vi "programacion 2 tercer parcial.vi"() -> ()   [LabVIEW 2011]
uses:
  Control programacion 2 tercer parcial.ctl
panel:
  out "Array":T1(array[cluster]) {"Velocidad 3" scale=0.0..180.0; "Velocidad 2" scale=0.0..180.0; "Velocidad1" scale=0.0..180.0}
  # "Se tiene que ingresar las tres velocidades de cada elemento del arreglo \nluego se debera de obtener el promedio de cada uno de los elementos del arreglo.\n\nIniciar arreglo, rellenar arreglo, obtener promedio, finalizar."
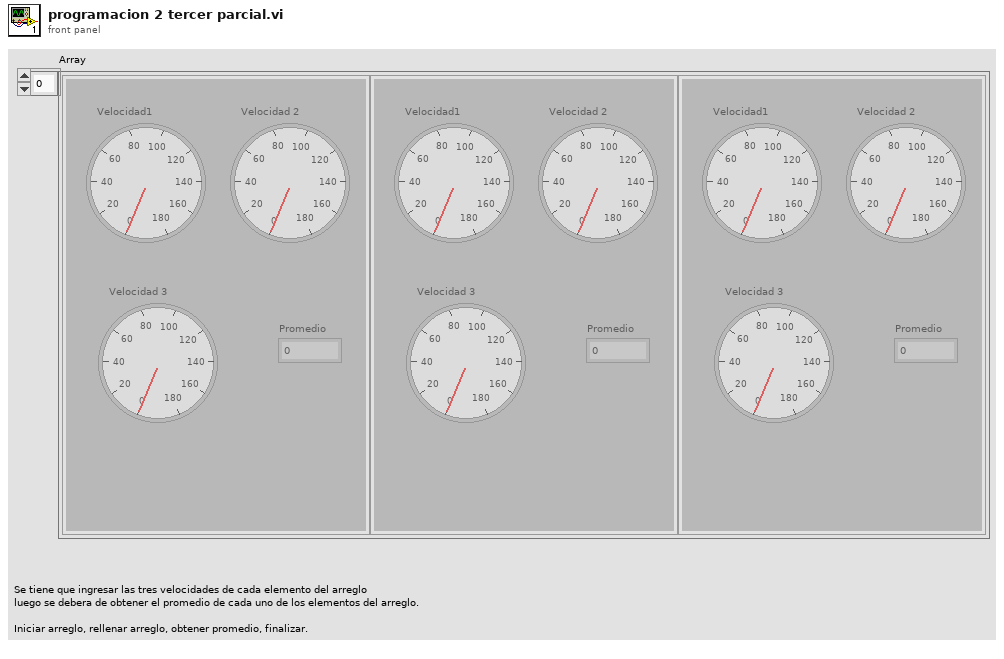
[diagram p1: front panel]
types:
  T1 = cluster{"Velocidad1":i32, "Velocidad 2":i32, "Velocidad 3":i32, "Promedio":dbl}[]
  T2 = typedef "Control programacion 2 tercer parcial.ctl" = enum16{"iniciar arreglo", "rellenar arreglo", "obtener promedio", "finalizar"}
  T3 = cluster{"Velocidad1":i32, "Velocidad 2":i32, "Velocidad 3":i32, "Promedio":dbl}
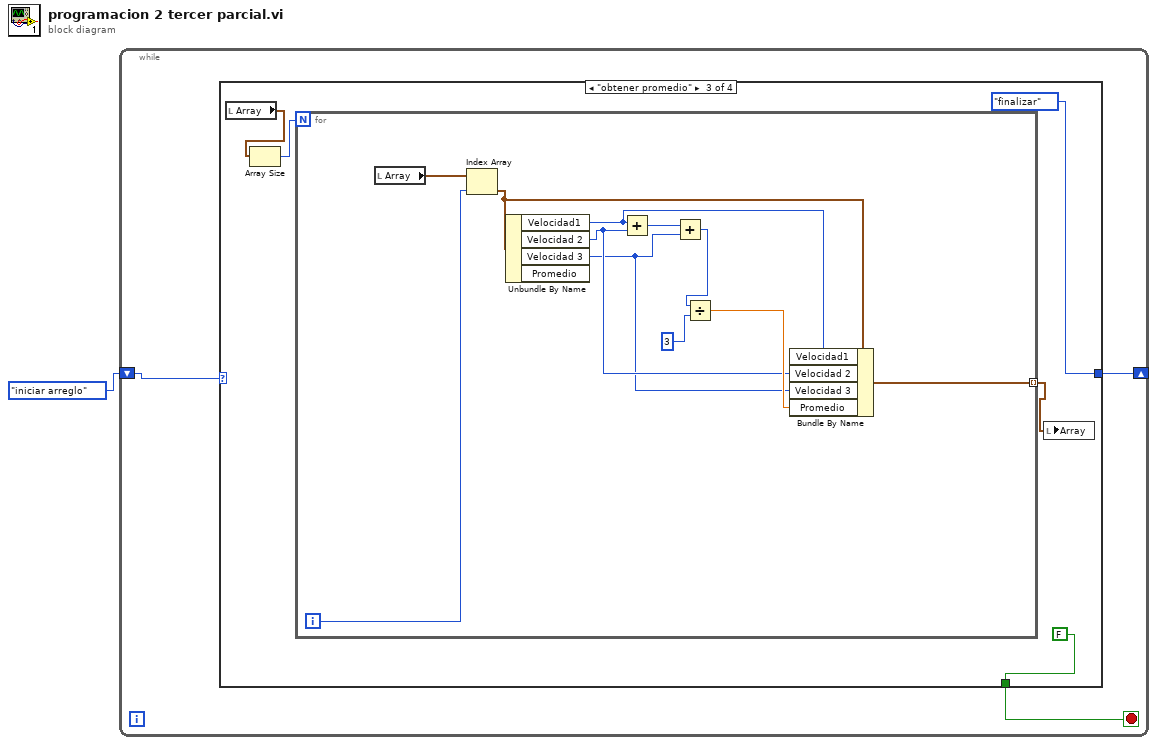
[diagram p0: block diagram]
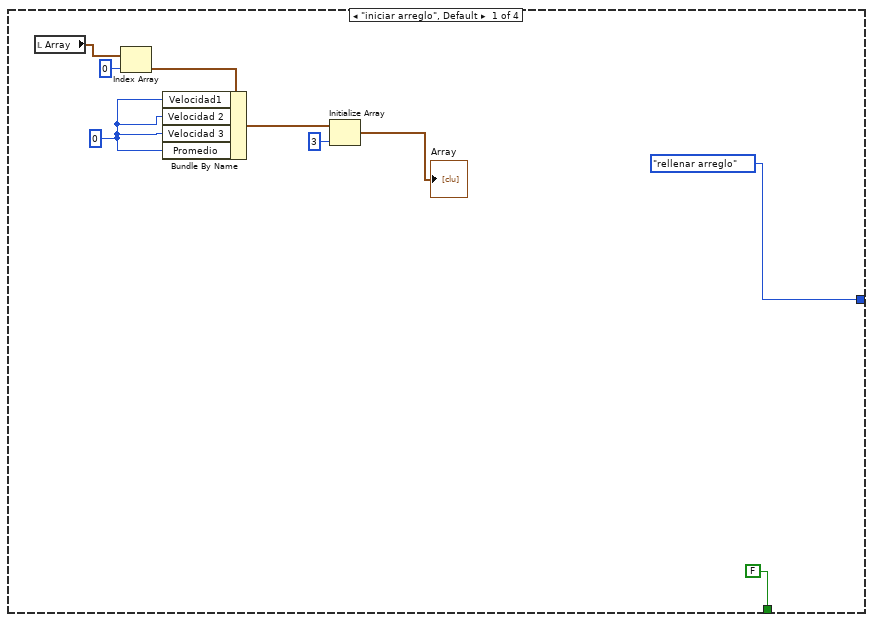
[diagram p2: hidden frame]
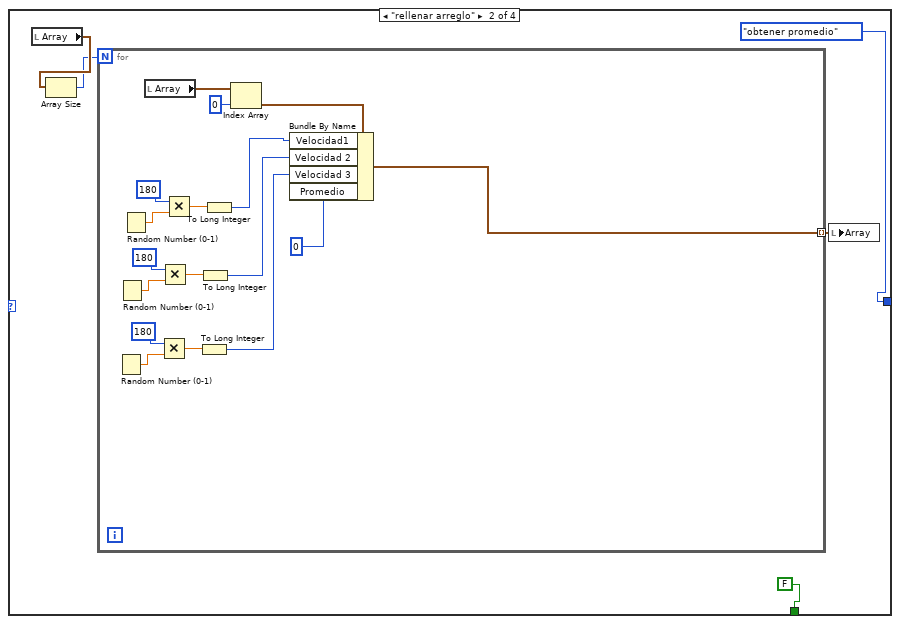
[diagram p3: hidden frame]
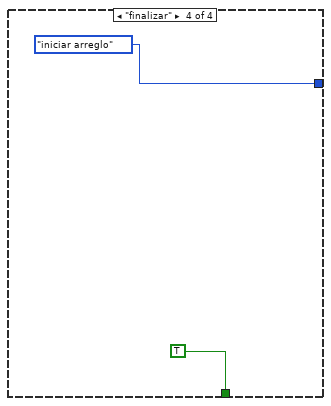
[diagram p4: hidden frame]
diagram:
  n1 = while {
    shift-right: [w3] -> _
    shift-left: Control_programacion_2_tercer_parcial."iniciar arreglo" -> [w4]
    stop <- w2 stop-if-true
    n2 = case shown="\"obtener promedio\"" w4 {
      tunnel: [Control_programacion_2_tercer_parcial."rellenar arreglo" Control_programacion_2_tercer_parcial."obtener promedio" Control_programacion_2_tercer_parcial."finalizar" Control_programacion_2_tercer_parcial."iniciar arreglo"] -> w3
      tunnel: [FALSE FALSE FALSE TRUE] -> w2
      frame "iniciar arreglo", Default {
        w10 = 0
        n3 = local read "Array"() -> (w13:T1)
        n4 = Index Array(array=w13, index=0) -> (element=w11:T3)
        n5 = Bundle By Name(cluster=w11, "Velocidad1"=w10, "Velocidad 2"=w10, "Velocidad 3"=w10, "Promedio"=w10) -> (w9:T3)
        n6 = Initialize Array(w9, 3 ("dimension size")) -> (→"Array":T1)
      }
      frame "rellenar arreglo" {
        n7 = local read "Array"() -> (w18:T1)
        n8 = Array Size(array=w18) -> (size(s)=w17:i32)
        n9 = for {
          N: w17 -> [_]
          tunnel: [w19] -> w16 mode=indexing
          n10 = Random Number (0-1)() -> (number: 0 to 1=w24:dbl)
          n11 = Random Number (0-1)() -> (number: 0 to 1=w26:dbl)
          n12 = Random Number (0-1)() -> (number: 0 to 1=w32:dbl)
          n13 = local read "Array"() -> (w35:T1)
          n14 = Multiply(x=180, y=w24) -> (x*y=w22:dbl)
          n15 = Multiply(x=180, y=w26) -> (x*y=w28:dbl)
          n16 = Multiply(x=180, y=w32) -> (x*y=w30:dbl)
          n17 = To Long Integer(number=w22) -> (32bit integer=w21:i32)
          n18 = To Long Integer(number=w28) -> (32bit integer=w25:i32)
          n19 = To Long Integer(number=w30) -> (32bit integer=w29:i32)
          n20 = Index Array(array=w35, index=0) -> (element=w33:T3)
          n21 = Bundle By Name(cluster=w33, "Velocidad1"=w29, "Velocidad 2"=w25, "Velocidad 3"=w21, "Promedio"=0) -> (w19:T3)
        }
        n22 = local write "Array"(w16) -> ()
      }
      frame "obtener promedio" {
        n23 = local read "Array"() -> (w40:T1)
        n24 = Array Size(array=w40) -> (size(s)=w39:i32)
        n25 = for {
          N: w39 -> [_]
          tunnel: [w46] -> w36 mode=indexing
          i -> [w42]
          n26 = local read "Array"() -> (w51:T1)
          n27 = Index Array(array=w51, index=w42) -> (element=w48:T3)
          n28 = Unbundle By Name(w48) -> ("Velocidad1"=w43:i32, "Velocidad 2"=w45:i32, "Velocidad 3"=w44:i32)  [unwired: 1 out]
          n29 = Add(x=w43, y=w45) -> (x+y=w50:i32)
          n30 = Add(x=w50, y=w44) -> (x+y=w49:i32)
          n31 = Divide(x=w49, y=3) -> (x/y=w47:dbl)
          n32 = Bundle By Name(cluster=w48, "Velocidad1"=w43, "Velocidad 2"=w45, "Velocidad 3"=w44, "Promedio"=w47) -> (w46:T3)
        }
        n33 = local write "Array"(w36) -> ()
      }
      frame "finalizar" {
      }
    }
  }
